vi "Get Scan Data Result OP30.vi"(8 "error in (no error)":errorcluster, 10 "RFID":string, 11 "Ref Out":T1 {"TS Parameter"."FCA" format="%01d"; "TS Parameter"."Target" min=1 max=100000; "TS Parameter"."PokaYoke" min=0 max=1}) -> (0 "error out":errorcluster, 2 "Table Control":string[][](array[string]), 3 "Ref Out 2":T1 {"TS Parameter"."FCA" format="%01d"; "TS Parameter"."Target" min=1 max=100000; "TS Parameter"."PokaYoke" min=0 max=1})   [LabVIEW 2020]
uses:
  Controls/TD SQL.ctl
  <vilib>/addons/database/Connection.llb/Conn ObjectReference.ctl
  Controls/WIP_State.ctl
  Controls/TS_Parameter.ctl
  <vilib>/addons/database/NI_Database_API.lvlib
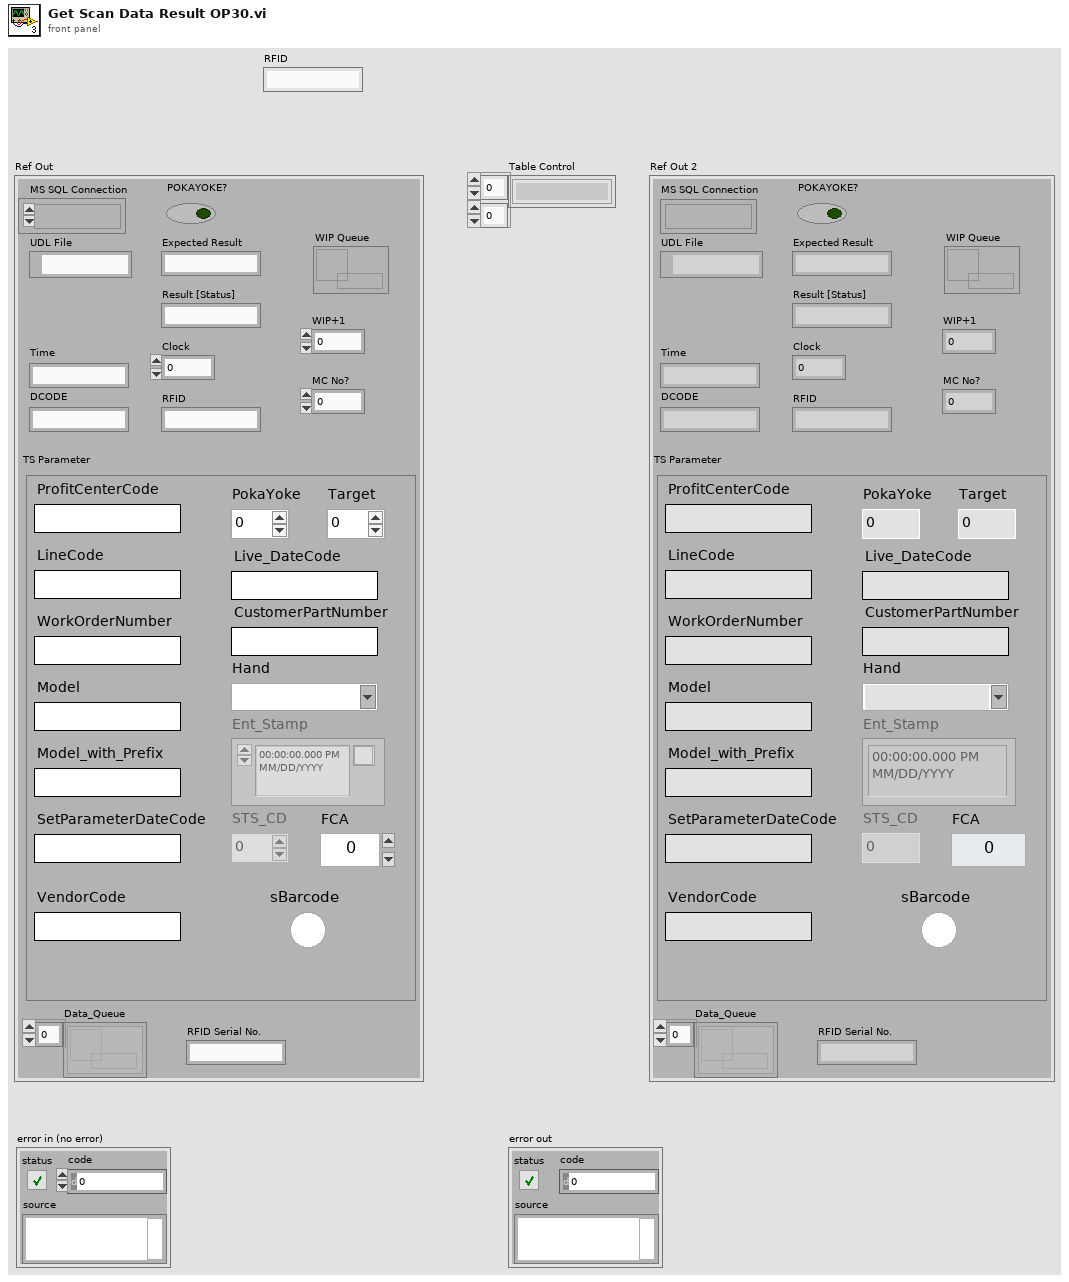
[diagram p1: front panel]
types:
  T1 = typedef "TD SQL.ctl" = cluster{"MS SQL Connection":T2, "UDL File":path, "Time":string, "DCODE":string, "WIP+1":i64, "MC No?":i32, "POKAYOKE?":bool, "Expected Result":string, "Result [Status]":string, "Clock":dbl, "RFID":string, "WIP Queue":refnum<queue>, "TS Parameter":T3, "Data_Queue":refnum<queue>[], "RFID Serial No.":string}
  T2 = typedef "NI_Database_API.lvlib/Conn ObjectReference.ctl" = refnum<k1>
  T3 = typedef "TS_Parameter.ctl" = cluster{"ProfitCenterCode":string, "LineCode":string, "WorkOrderNumber":string, "Model":string, "Model_with_Prefix":string, "VendorCode":string, "SetParameterDateCode":string, "PokaYoke":i32, "Target":i32, "Live_DateCode":string, "CustomerPartNumber":string, "Hand":string, "sBarcode":bool, "FCA":i32, "Ent_Stamp":timestamp, "STS_CD":dbl}
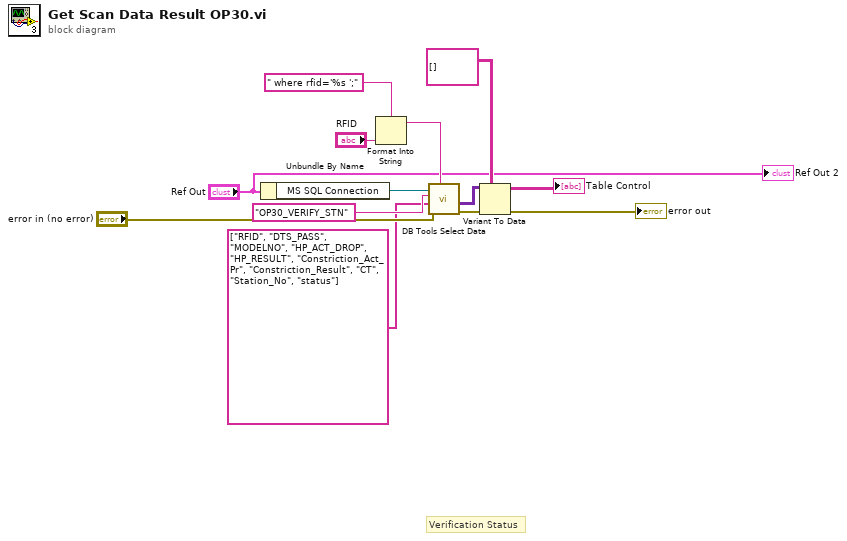
[diagram p0: block diagram]
diagram:
  # "Verification Status"
  n1 = Unbundle By Name("Ref Out") -> ("MS SQL Connection"=w5:T2)
  n2 = Format Into String(format string=" where rfid='%s ';" ("condition"), "RFID") -> (resulting string=w4:string)  [unwired: 2 in, 1 out]
  n3 = call <vilib>:"DB Tools Select Data.vi"("condition"=w4, "error in (no error)"="error in (no error)", "columns"=string[] ["RFID", "DTS_PASS", "MODELNO", "HP_ACT_DROP", "HP_RESULT", "Constriction_Act_Pr", "Constriction_Result", "CT", "Station_No", "status"], "table"="OP30_VERIFY_STN", "connection reference"=w5) -> ("error out"=w10:errorcluster, "data"=w9:variant[][])  [unwired: 1 in, 1 out]
  n4 = Variant To Data(error in=w10, type=string[][] [] ("Table Control"), Variant=w9) -> (data=→"Table Control":string[][], error out=→"error out":errorcluster)
  "Ref Out 2" <- "Ref Out"
